vi "TDMS_Write.vi"(2 "namesArray":string[](array[string])=["Cx", "Cy", "I0x", "mux", "wx", "i1x", "I0y", "muy", "I1y"], 3 "Array - Numeric":dbl[](array[numeric]), 4 "groupName":string="beamData", 5 "TDMS_HandleIn":refnum<k34>) -> (0 "errorTDMS_Write":errorcluster, 1 "TDMS_HandleOut":refnum<k34>)   [LabVIEW 2021]
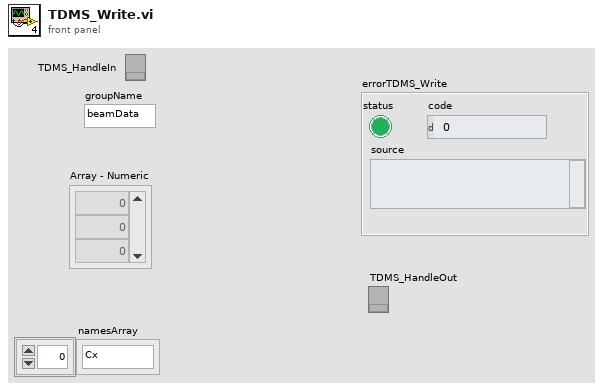
[diagram p1: front panel]
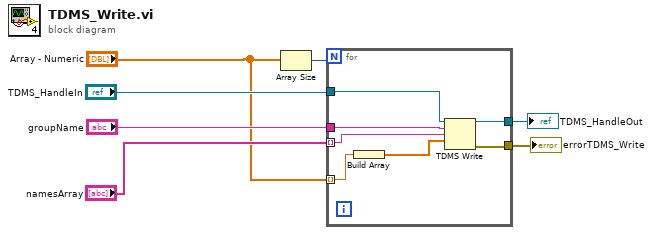
[diagram p0: block diagram]
diagram:
  n1 = Array Size(array="Array - Numeric") -> (size(s)=w2:i32)
  n2 = for {
    N: w2 -> [_]
    tunnel: "TDMS_HandleIn" -> [w14]
    tunnel: "groupName" -> [w13]
    tunnel: "namesArray" -> [w8] mode=indexing
    tunnel: [w12] -> w7
    tunnel: "Array - Numeric" -> [w10] mode=indexing
    tunnel: [w11] -> w5
    n3 = Build Array(w10) -> (w9:dbl[])
    n4 = TDMS Write(0:w14, 5:w13, 7:w8, 9:w9) -> (4:w11:refnum<k34>, 15:w12:errorcluster)  [unwired: 2 in, 2 out]
  }
  "errorTDMS_Write" <- w7
  "TDMS_HandleOut" <- w5
